vi "PH_Beckhoff_PPMA-Rods.contents.vi"   [LabVIEW 2014, in "PH_Beckhoff_PPMA-Rods.lvlib"]
doc: "This class is forseen to xxx\n\nThis class is part of the PHELIX xxx layer."
uses:
  PH_Beckhoff_PPMA-Rods.lvlib
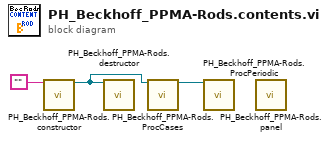
[diagram p0: block diagram]
diagram:
  n1 = call "PH_Beckhoff_PPMA-Rods.constructor.vi"("name"="") -> ("i ref out"=w1:refnum<vi>)  [unwired: 16 in, 2 out]
  n2 = call "PH_Beckhoff_PPMA-Rods.destructor.vi"("i ref in"=w1) -> ()  [unwired: 18 in, 1 out]
  n3 = call "PH_Beckhoff_PPMA-Rods.ProcCases.vi"("i ref in"=w1) -> ("i ref out"=w2:refnum<vi>)  [unwired: 16 in, 2 out]
  n4 = call "PH_Beckhoff_PPMA-Rods.ProcPeriodic.vi"("i ref in"=w2) -> ()  [unwired: 16 in, 3 out]
  n5 = call "PH_Beckhoff_PPMA-Rods.panel.vi"() -> ()  [unwired: 19 in, 1 out]
